vi "Update DO status.vi"(7 "Homing?":bool, 8 "error in (no error)":errorcluster, 11 "ES array":bool[](array[boolean])) -> (0 "error out":errorcluster, 3 "Motor control out":T1, 5 "Home?":bool)   [LabVIEW 2020]
uses:
  controls/Motor FGV states ---typedef.ctl
  Controls/Motor controls---typedef.ctl
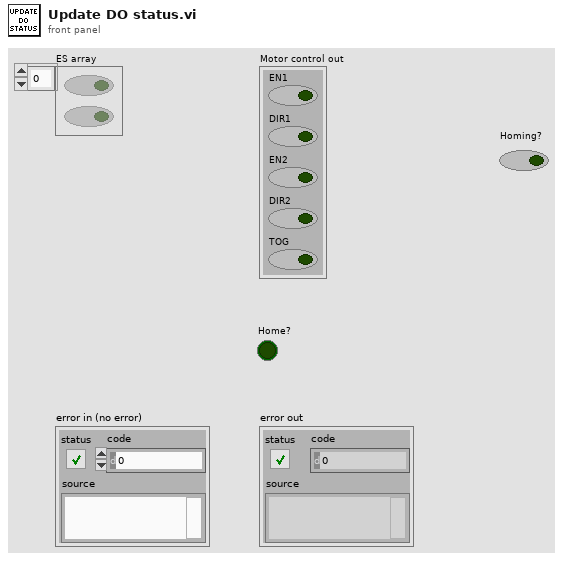
[diagram p1: front panel]
types:
  T1 = typedef "Motor controls---typedef.ctl" = cluster{"EN1":bool, "DIR1":bool, "EN2":bool, "DIR2":bool, "TOG":bool}
  T2 = typedef "Motor FGV states ---typedef.ctl" = enum16{"Set", "Reset", "Get"}
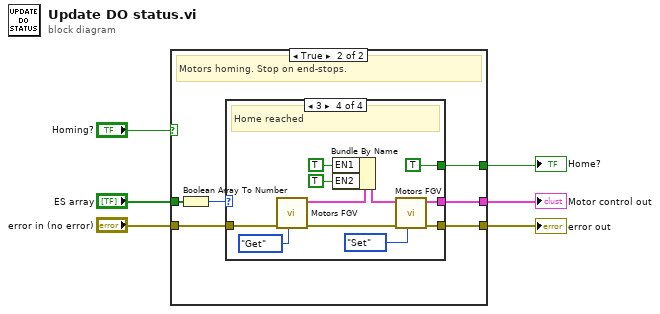
[diagram p0: block diagram]
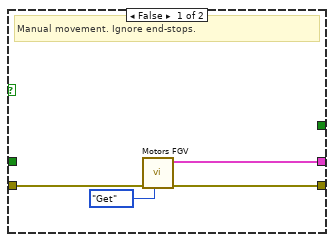
[diagram p2: hidden frame]
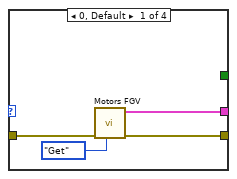
[diagram p3: hidden frame]
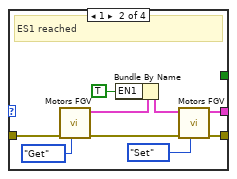
[diagram p4: hidden frame]
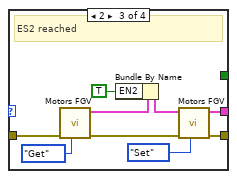
[diagram p5: hidden frame]
diagram:
  n1 = case shown="True" "Homing?" {
    tunnel: [w8 w16] -> w6
    tunnel: [w9 w15] -> w5
    tunnel: "error in (no error)" -> [w10 w14]
    tunnel: "ES array" -> [_ w12]
    tunnel: [_ w11] -> w2
    frame False {
      # "Manual movement. Ignore end-stops."
      n2 = call "Motors FGV.vi"("Action"=Motor_FGV_states_---typedef."Get", "error in (no error)"=w10) -> ("error out"=w9:errorcluster, "Motor control out"=w8:T1)  [unwired: 8 in]
    }
    frame True {
      # "Motors homing. Stop on end-stops."
      n3 = Boolean Array To Number(Boolean array=w12) -> (number=w13:u32)
      n4 = case shown="3" w13 {
        tunnel: w14 -> [w20 w29 w38 w49]
        tunnel: [w19 w23 w32 w43] -> w15
        tunnel: [w18 w21 w30 w41] -> w16
        tunnel: [_ _ _ TRUE] -> w11
        frame 0, Default {
          n5 = call "Motors FGV.vi"("Action"=Motor_FGV_states_---typedef."Get", "error in (no error)"=w20) -> ("error out"=w19:errorcluster, "Motor control out"=w18:T1)  [unwired: 8 in]
        }
        frame 1 {
          # "ES1 reached"
          n6 = call "Motors FGV.vi"("Action"=Motor_FGV_states_---typedef."Get", "error in (no error)"=w29) -> ("error out"=w25:errorcluster, "Motor control out"=w27:T1)  [unwired: 8 in]
          n7 = Bundle By Name(cluster=w27, "EN1"=TRUE) -> (w24:T1)
          n8 = call "Motors FGV.vi"("Action"=Motor_FGV_states_---typedef."Set", "error in (no error)"=w25, "Motor control in"=w24) -> ("error out"=w23:errorcluster, "Motor control out"=w21:T1)  [unwired: 7 in]
        }
        frame 2 {
          # "ES2 reached"
          n9 = call "Motors FGV.vi"("Action"=Motor_FGV_states_---typedef."Get", "error in (no error)"=w38) -> ("error out"=w34:errorcluster, "Motor control out"=w36:T1)  [unwired: 8 in]
          n10 = Bundle By Name(cluster=w36, "EN2"=TRUE ("EN1")) -> (w33:T1)
          n11 = call "Motors FGV.vi"("Action"=Motor_FGV_states_---typedef."Set", "error in (no error)"=w34, "Motor control in"=w33) -> ("error out"=w32:errorcluster, "Motor control out"=w30:T1)  [unwired: 7 in]
        }
        frame 3 {
          # "Home reached"
          n12 = call "Motors FGV.vi"("Action"=Motor_FGV_states_---typedef."Get", "error in (no error)"=w49) -> ("error out"=w45:errorcluster, "Motor control out"=w47:T1)  [unwired: 8 in]
          n13 = Bundle By Name(cluster=w47, "EN1"=TRUE, "EN2"=TRUE ("EN1")) -> (w44:T1)
          n14 = call "Motors FGV.vi"("Action"=Motor_FGV_states_---typedef."Set", "error in (no error)"=w45, "Motor control in"=w44) -> ("error out"=w43:errorcluster, "Motor control out"=w41:T1)  [unwired: 7 in]
        }
      }
    }
  }
  "Motor control out" <- w6
  "error out" <- w5
  "Home?" <- w2
